vi "DB_Select Data.vi"(7 "condition":string, 8 "error in (no error)":errorcluster, 9 "columns":string[](array[string]), 10 "table":string, 11 "connection reference":T1) -> (0 "error out":errorcluster, 3 "data":string[][](array[string]))   [LabVIEW 2017]
uses:
  <vilib>/addons/database/Connection.llb/Conn ObjectReference.ctl
  <vilib>/addons/database/_DB Variant To Data/Database Variant To Data.xnode
  <vilib>/addons/database/NI_Database_API.lvlib
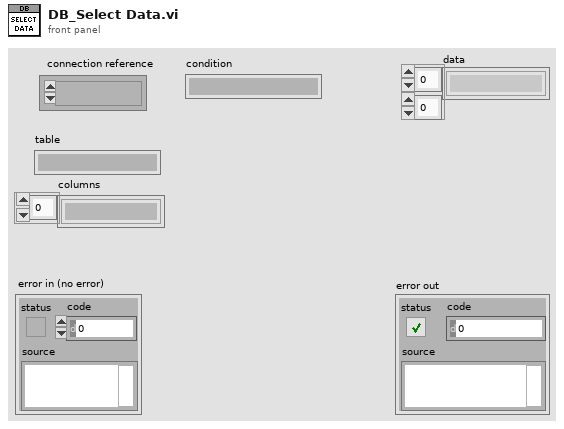
[diagram p1: front panel]
types:
  T1 = typedef "NI_Database_API.lvlib/Conn ObjectReference.ctl" = refnum<k1>
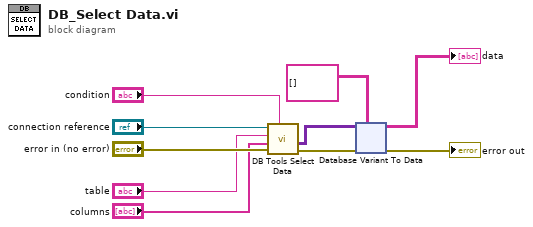
[diagram p0: block diagram]
diagram:
  n1 = call <vilib>:"DB Tools Select Data.vi"("condition"="condition", "error in (no error)"="error in (no error)", "columns"="columns", "table"="table", "connection reference"="connection reference") -> ("error out"=w10:errorcluster, "data"=w9:variant[][])  [unwired: 1 in, 1 out]
  n2 = xnode "Database Variant To Data"("database variant"=w9, "error in (no error)"=w10, "type"=string[][] []) -> ("data"=→"data":string[][], "error out"=→"error out":errorcluster)
